vi "SetVariantAttributes.vi"(1 "values":variant[](array[variant]), 2 "names":string[](array[string]), 3 "Variant In":variant) -> (0 "Variant Out":variant)   [LabVIEW 2014]
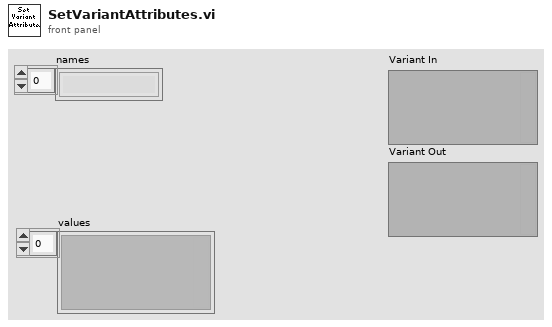
[diagram p1: front panel]
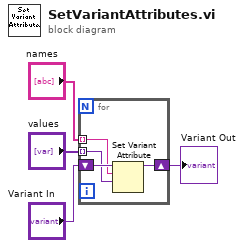
[diagram p0: block diagram]
diagram:
  n1 = for {
    shift-right: [w8] -> w1
    shift-left: "Variant In" -> [w7]
    tunnel: "names" -> [w6] mode=indexing
    tunnel: "values" -> [w5] mode=indexing
    n2 = Set Variant Attribute(Variant=w7, name=w6, value=w5) -> (Variant out=w8:variant)  [unwired: 1 in, 2 out]
  }
  "Variant Out" <- w1
